vi "登录对话框.vi"() -> (1 "输出":bool, 2 "序列号":string, 3 "串口号":refnum<visa-resource-name>="COM4")   [LabVIEW 2016, in "斯坦道CODMn.lvlib"]
uses:
  <vilib>/Utility/miscctls.llb/LVPointTypeDef.ctl
panel:
  in  "取消":bool
  in  "确定":bool
  in  "序列号":string
  in  "VISA resource name":refnum<visa-resource-name>="COM4" caption="串口号"
  # "请选择串口号和输入序列号"
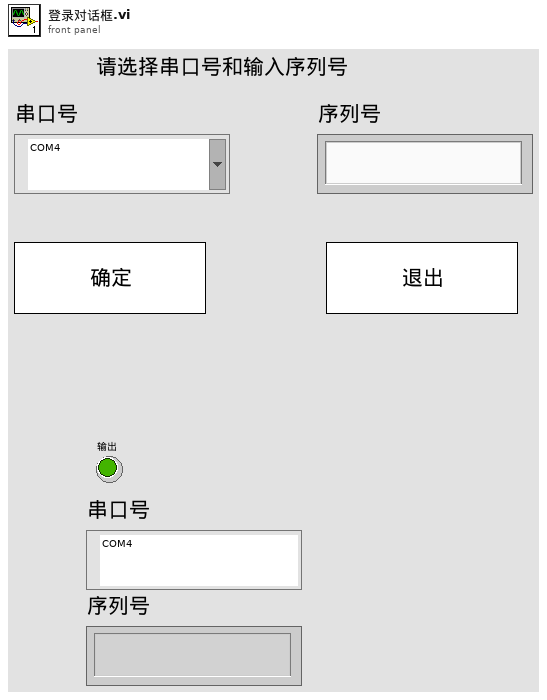
[diagram p1: front panel]
types:
  T1 = typedef "LVPointTypeDef.ctl" = cluster{"Horizontal":i16, "Vertical":i16}
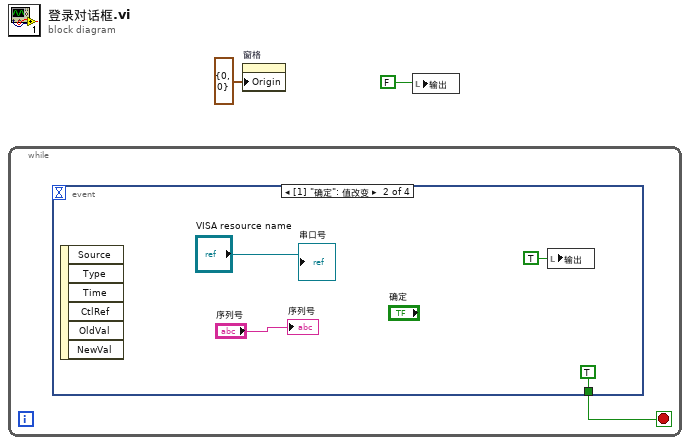
[diagram p0: block diagram]
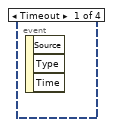
[diagram p2: hidden frame]
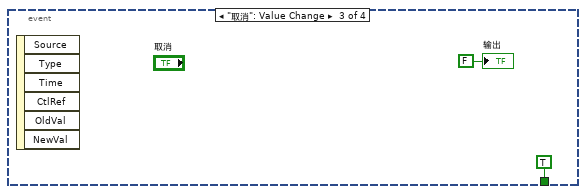
[diagram p3: hidden frame]
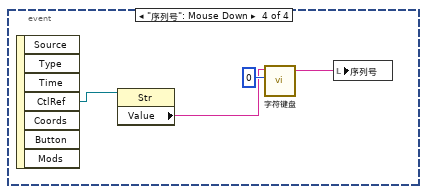
[diagram p4: hidden frame]
diagram:
  n1 = while {
    stop <- w3 stop-if-true
    n2 = event shown="[1] \"确定\": 值改变" {
      selector: _ -> [_ _ _ _]
      dyn-events: _ -> [_ _ _ _]
      timeout: _ -> [_ _ _ _]
      tunnel: [_ TRUE ("确定") TRUE ("确定") _] -> w3
      event Timeout {
        n3 = event-data() -> ()  [unwired: 1 in, 3 out]
      }
      event "确定": Value Change {
        n4 = event-data() -> ()  [unwired: 1 in, 6 out]
        n5 = local write "输出"(TRUE ("输出")) -> ()
        "串口号" <- "VISA resource name"
        "序列号" <- "序列号"
      }
      event "取消": Value Change {
        n6 = event-data() -> ()  [unwired: 1 in, 6 out]
        "输出" <- FALSE ("输出")
      }
      event "序列号": Mouse Down {
        n7 = event-data() -> ("CtlRef"=w11:refnum<vi>)  [unwired: 1 in, 6 out]
        n8 = property class="Str"(reference=w11) -> ("Value"=w10:string)  [unwired: 1 in, 2 out]
        n9 = call "字符键盘.vi"("显示样式"=u32 0, "原值"=w10) -> ("x+y"=w12:string)  [unwired: 9 in]
        n10 = local write "序列号"(w12) -> ()
      }
    }
  }
  n11 = property on="窗格" class="Pane"("Origin"=T1 {"Horizontal"=0, "Vertical"=0} ("原点")) -> ()  [unwired: 2 in, 2 out]
  n12 = local write "输出"(FALSE ("输出")) -> ()
